vi "TCP UDP Reference FGV.vi"(7 "Command":T1=enum."Get", 8 "Error In":errorcluster, 9 "UDP Connection ID":refnum<k16>, 10 "TCP Listener ID":refnum<k5>, 11 "TCP Connection ID":refnum<k5>) -> (0 "Error Out":errorcluster, 1 "UDP Connection ID":refnum<k16>, 2 "TCP Connection ID":refnum<k5>, 3 "TCP Listener ID":refnum<k5>)   [LabVIEW 2017, in "Game.lvlib" / "GameComms.lvlib"]
uses:
  GameComms.lvlib
  TypeDefs/TCP UDP Ref FGV Commands.ctl
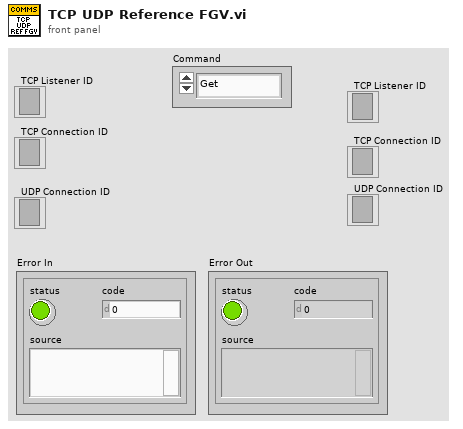
[diagram p1: front panel]
types:
  T1 = typedef "Game.lvlib/GameComms.lvlib/TCP UDP Ref FGV Commands.ctl" = enum16{"Set", "Get"}
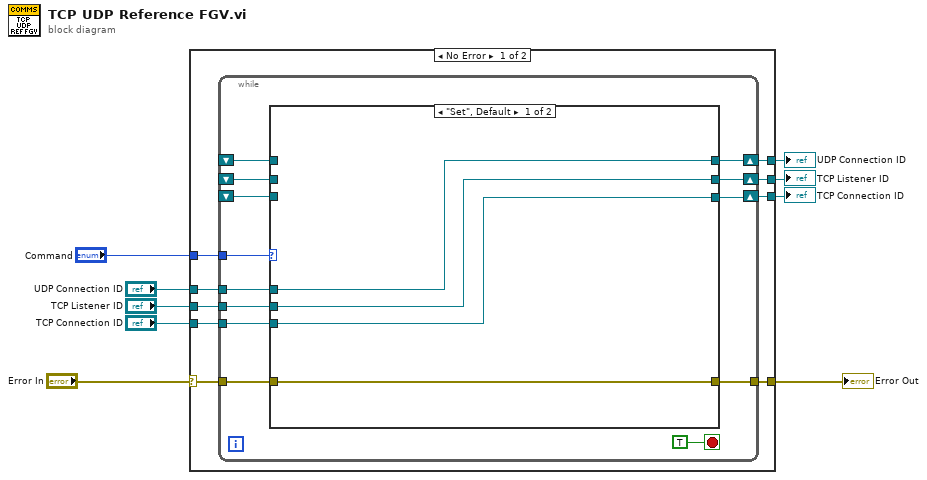
[diagram p0: block diagram]
diagram:
  n1 = case shown="No Error" "Error In" {
    selector: "Error In" -> [w17 w40]
    tunnel: [w13 w40] -> w8
    tunnel: "Command" -> [w18 _]
    tunnel: "UDP Connection ID" -> [w16 _]
    tunnel: "TCP Listener ID" -> [w15 _]
    tunnel: "TCP Connection ID" -> [w14 _]
    tunnel: [w12 _] -> w3
    tunnel: [w11 _] -> w2
    tunnel: [w10 _] -> w1
    frame No Error {
      n2 = while {
        tunnel: w18 -> [w30]
        tunnel: w17 -> [w29]
        tunnel: w16 -> [w28]
        tunnel: w15 -> [w27]
        tunnel: w14 -> [w26]
        shift-right: [w23] -> w10
        shift-left: _ -> [w20]
        shift-right: [w24] -> w11
        shift-left: _ -> [w21]
        shift-right: [w25] -> w12
        shift-left: _ -> [w22]
        tunnel: [w19] -> w13
        stop <- TRUE stop-if-true
        n3 = case shown="\"Set\", Default" w30 {
          tunnel: w29 -> [w32 w36]
          tunnel: w28 -> [w35 _]
          tunnel: w27 -> [w34 _]
          tunnel: w26 -> [w33 _]
          tunnel: [w35 w39] -> w25
          tunnel: [w34 w38] -> w24
          tunnel: [w33 w37] -> w23
          tunnel: w22 -> [_ w39]
          tunnel: w21 -> [_ w38]
          tunnel: w20 -> [_ w37]
          tunnel: [w32 w36] -> w19
          frame "Set", Default {
          }
          frame "Get" {
          }
        }
      }
    }
    frame Error {
    }
  }
  "Error Out" <- w8
  "UDP Connection ID" <- w3
  "TCP Listener ID" <- w2
  "TCP Connection ID" <- w1
